vi "TurnBarrelsLimit.vi"   [LabVIEW 2014]
types:
  T1 = typedef "WPI_SwitchDevRef.ctl" = cluster{"DevStatus":errorcluster, "DIO Channel":T2, "Controller":T3, "CntIndex":T4, "Normally Closed":bool}
  T2 = typedef "FPGA_DIOChannel.ctl" = enum8{"DIO 0", "DIO 1", "DIO 2", "DIO 3", "DIO 4", "DIO 5", "DIO 6", "DIO 7", "DIO 8", "DIO 9", "DIO MXP 0", "DIO MXP 1", "DIO MXP 2", "DIO MXP 3", "DIO MXP 4", "DIO MXP 5", "DIO MXP 6", "DIO MXP 7", "DIO MXP 8", "DIO MXP 9", "DIO MXP 10", "DIO MXP 11", "DIO MXP 12", "DIO MXP 13", "DIO MXP 14", "DIO MXP 15", "Invalid"}
  T3 = typedef "FPGA_TypedefDigitalModule.ctl" = enum16{"Controller 1"}
  T4 = typedef "FPGA_CounterCtrSystemIndex.ctl" = enum8{"Ctr 0", "Ctr 1", "Ctr 2", "Ctr 3", "Ctr 4", "Ctr 5", "Ctr 6", "Ctr 7", "Invalid"}
  T5 = typedef "WPI_MotorControlDeviceRef.ctl" = cluster{"DeviceStatus":errorcluster, "Type":T6, "PWM":cluster{"Controller":T3, "PWM Channel":T7, "DeadBand":T8}, "CAN":cluster{"Device Number":u8, "Control Mode":T9, "Semaphore":T10, "Max Vout":dbl, "TalonSRX Control Mode":T11}, "Invert":bool, "TransformRef":T12, "InvTransformRef":T12}
  T6 = typedef "WPI_MotorControlType.ctl" = enum16{"PWM", "CAN", "CANTalonSRX"}
  T7 = typedef "FPGA_DIOPWMChannel.ctl" = enum8{"PWM 0", "PWM 1", "PWM 2", "PWM 3", "PWM 4", "PWM 5", "PWM 6", "PWM 7", "PWM 8", "PWM 9", "PWM MXP 0", "PWM MXP 1", "PWM MXP 2", "PWM MXP 3", "PWM MXP 4", "PWM MXP 5", "PWM MXP 6", "PWM MXP 7", "PWM MXP 8", "PWM MXP 9", "Invalid"}
  T8 = typedef "WPI_PWMDeadband.ctl" = cluster{"Name":string, "maxPositivePwm":i32, "minPositivePwm":i32, "centerPwm":i32, "maxNegativePwm":i32, "minNegativePwm":i32, "angularRange":u16}
  T9 = typedef "WPI_CANJaguar_ControlMode.ctl" = enum8{"Percent VBus", "Current", "Speed", "Position", "Voltage"}
  T10 = typedef "Semaphore RefNum" = refnum<k1>
  T11 = typedef "WPI_CANTalonSRX_APIControlMode.ctl" = enum8{"Percent VBus", "Speed", "Position", "Slave", "Unchanged / Invalid"}
  T12 = typedef "WPI_PWMTransform_ConPane.ctl" = refnum<vi>
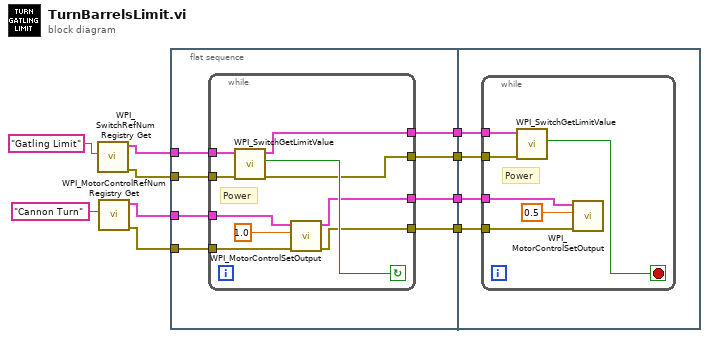
[diagram p0: block diagram]
diagram:
  n1 = call <vilib>:"WPI_SwitchRefNum Registry Get.vi"("refnum name"="Gatling Limit") -> ("error out"=w7:errorcluster, "SwitchDevRef"=w8:T1)  [unwired: 9 in]
  n2 = call <vilib>:"WPI_MotorControlRefNum Registry Get.vi"("refnum name"="Cannon Turn") -> ("error out"=w5:errorcluster, "MotorControlDevRef"=w6:T5)  [unwired: 9 in]
  n3 = flat-sequence {
    tunnel: w8 -> [w18]
    tunnel: w7 -> [w17]
    tunnel: w6 -> [w16]
    tunnel: w5 -> [w15]
    tunnel: [w14] -> w4
    tunnel: [w13] -> w3
    tunnel: [w12] -> w2
    tunnel: [w11] -> w1
    tunnel: w4 -> [w32]
    tunnel: w3 -> [w31]
    tunnel: w2 -> [w30]
    tunnel: w1 -> [w29]
    frame #0 {
      n4 = while {
        tunnel: w18 -> [w28]
        tunnel: w17 -> [w27]
        tunnel: w16 -> [w25]
        tunnel: w15 -> [w24]
        tunnel: [w22] -> w14
        tunnel: [w21] -> w13
        tunnel: [w20] -> w12
        tunnel: [w19] -> w11
        stop <- w23 continue-if-true
        # "Power"
        n5 = call <vilib>:"WPI_SwitchGetLimitValue.vi"("error in (no error)"=w27, "SwitchDevRef"=w28) -> ("error out"=w21:errorcluster, "Switch Pressed"=w23:bool, "SwitchDevRef"=w22:T1)  [unwired: 7 in]
        n6 = call <vilib>:"WPI_MotorControlSetOutput.vi"("error in (no error)"=w24, "Output"=1.0, "MotorControlDevRef"=w25) -> ("error out"=w20:errorcluster, "MotorControlDevRef"=w19:T5)  [unwired: 6 in, 1 out]
      }
    }
    frame #1 {
      n7 = while {
        tunnel: w32 -> [w37]
        tunnel: w31 -> [w36]
        tunnel: w30 -> [w35]
        tunnel: w29 -> [w34]
        stop <- w33 stop-if-true
        # "Power"
        n8 = call <vilib>:"WPI_SwitchGetLimitValue.vi"("error in (no error)"=w36, "SwitchDevRef"=w37) -> ("Switch Pressed"=w33:bool)  [unwired: 7 in, 2 out]
        n9 = call <vilib>:"WPI_MotorControlSetOutput.vi"("error in (no error)"=w35, "Output"=0.5, "MotorControlDevRef"=w34) -> ()  [unwired: 6 in, 3 out]
      }
    }
  }
